vi "Meas Result Generate TWM InpZ Correction - Process Measurement.vi"(7 "table ref":refnum<vi>, 8 "error in":errorcluster, 11 "meas":T3={"swp cfg"={"N"=0, "R"=0, "f list"=[], "smpl delay"=0.0, "set delay"=0.0, "set delay np"=0.0, "meas root"=path "", "meas name"="", "meas a-index"=FALSE, "rnd sweep"=FALSE, "mode"=enum."Frequency", "swp mode"=enum."Linear", "avg"=0, "subrec"=0, "multi-freq"=FALSE, "selfcal"=FALSE, "selfcal period [h]"=0.0}, "bridge"={"type"=enum."TWM client", "TWM"={"pipe name"="", "parameters"=[], "handle"=0, "fixed aper [s]"=0.0, "f-list [Hz]"=[], "discrete f-list"=FALSE, "unc mode"=enum."None", "unc mcc"=0, "unc first"=FALSE, "alg id"=enum."TWM-LowZ - Low Z measurement"}, "last f"=0.0, "bias comp"={"bias type"=enum."dummy", "VISA"="", "Enable"=FALSE, "channel qu"=[], "channel Uinit"=[]}, "sim mode"=enum."Generic RLC network", "channel idns"=[], "sim phases"=1}, "src"={"type"=enum."Tektronix AFG3101C", "afg"={"VISA"="", "const"=0.0, "gen DC"=FALSE, "ext ref"=FALSE}, "cDAQ dds"={"device"="", "channels"=[], "mclk source"="", "mclk [Hz]"=0.0, "fs [Hz]"=0.0, "block [s]"=0.0, "buf [s]"=0.0, "task"="", "cmd queue"=refnum, "proc ref"=refnum, "smpl clock out"="/cDAQ3/PFI0", "export smpl clock"=FALSE, "DC ofs [V]"=[], "timebase source"="", "timebase mode"=enum."Local", "dither"=enum."Disabled", "dither level"=0.0}, "gain [V/A]"=1.0, "F5xxx session"={"VISA"="", "mode"=enum."AC voltage", "Earth on"=FALSE, "Ext ref lock"=FALSE}}, "results"=refnum} {"src"."cDAQ dds"."channels" min=0 step=1; "bridge"."TWM"."f-list [Hz]" format="%#_6p"; "swp cfg"."f list"."bias" format="%#_3p"; "swp cfg"."f list"."level" format="%#_3p"; "swp cfg"."f list"."fs [Hz]" format="%#_5p"; "swp cfg"."f list"."time [s]" format="%#_3p"; "swp cfg"."f list"."f/fs" format="%#_3p"; "swp cfg"."f list"."periods" format="%#_3f"; "swp cfg"."f list"."f [Hz]" format="%#_5p"}) -> (0 "error out":errorcluster, 3 "correction data":T1)   [LabVIEW 2020]
doc: "Generates input impedance correction matrix for TWM."
uses:
  meas session.ctl
  Meas Sweep Config.ctl
  Meas Freq Info.ctl
  meas_swp_mode.ctl
  meas_sweep_flist_mode.ctl
  bridge/Bridge Session.ctl
  bridge/Bridge Type.ctl
  drivers/TWM client/TWM Session.ctl
  drivers/TWM client/TWM parameters.ctl
  drivers/TWM client/Meas Proc QWTB Uncertainty Mode.ctl
  bridge/Bridge Algorithm.ctl
  bridge/Bridge Bias Session.ctl
  bridge/Bridge Bias Type.ctl
  bridge/Bridge Sim Mode.ctl
  source/Source Session.ctl
  source/Source Type.ctl
  drivers/AFG3101C/AFG3101C Session.ctl
  drivers/cDAQ DDS/cDAQ DDS Session.ctl
  drivers/cDAQ DDS/cDAQ DDS Setup.ctl
  drivers/cDAQ DDS/cDAQ DDS Timebase Mode.ctl
  drivers/cDAQ DDS/cDAQ DDS Dither.ctl
  drivers/Fluke 5XXX/top_lev/F5xxx_session.ctl
  drivers/Fluke 5XXX/top_lev/F5xxx_output_mode.ctl
  Meas Results Ref.ctl
  Meas Results.ctl
  bridge/Bridge Frequency Readings Data.ctl
  drivers/TWM client/Meas Proc QWTB Spectrum Data.ctl
  drivers/TWM client/TWM Phase Info.ctl
  Meas Results TWM Digitizer Correction Data.ctl
  Meas Results Correction Structuring Mode.ctl
  Meas Results Sweep Data Uncertainty Mode.ctl
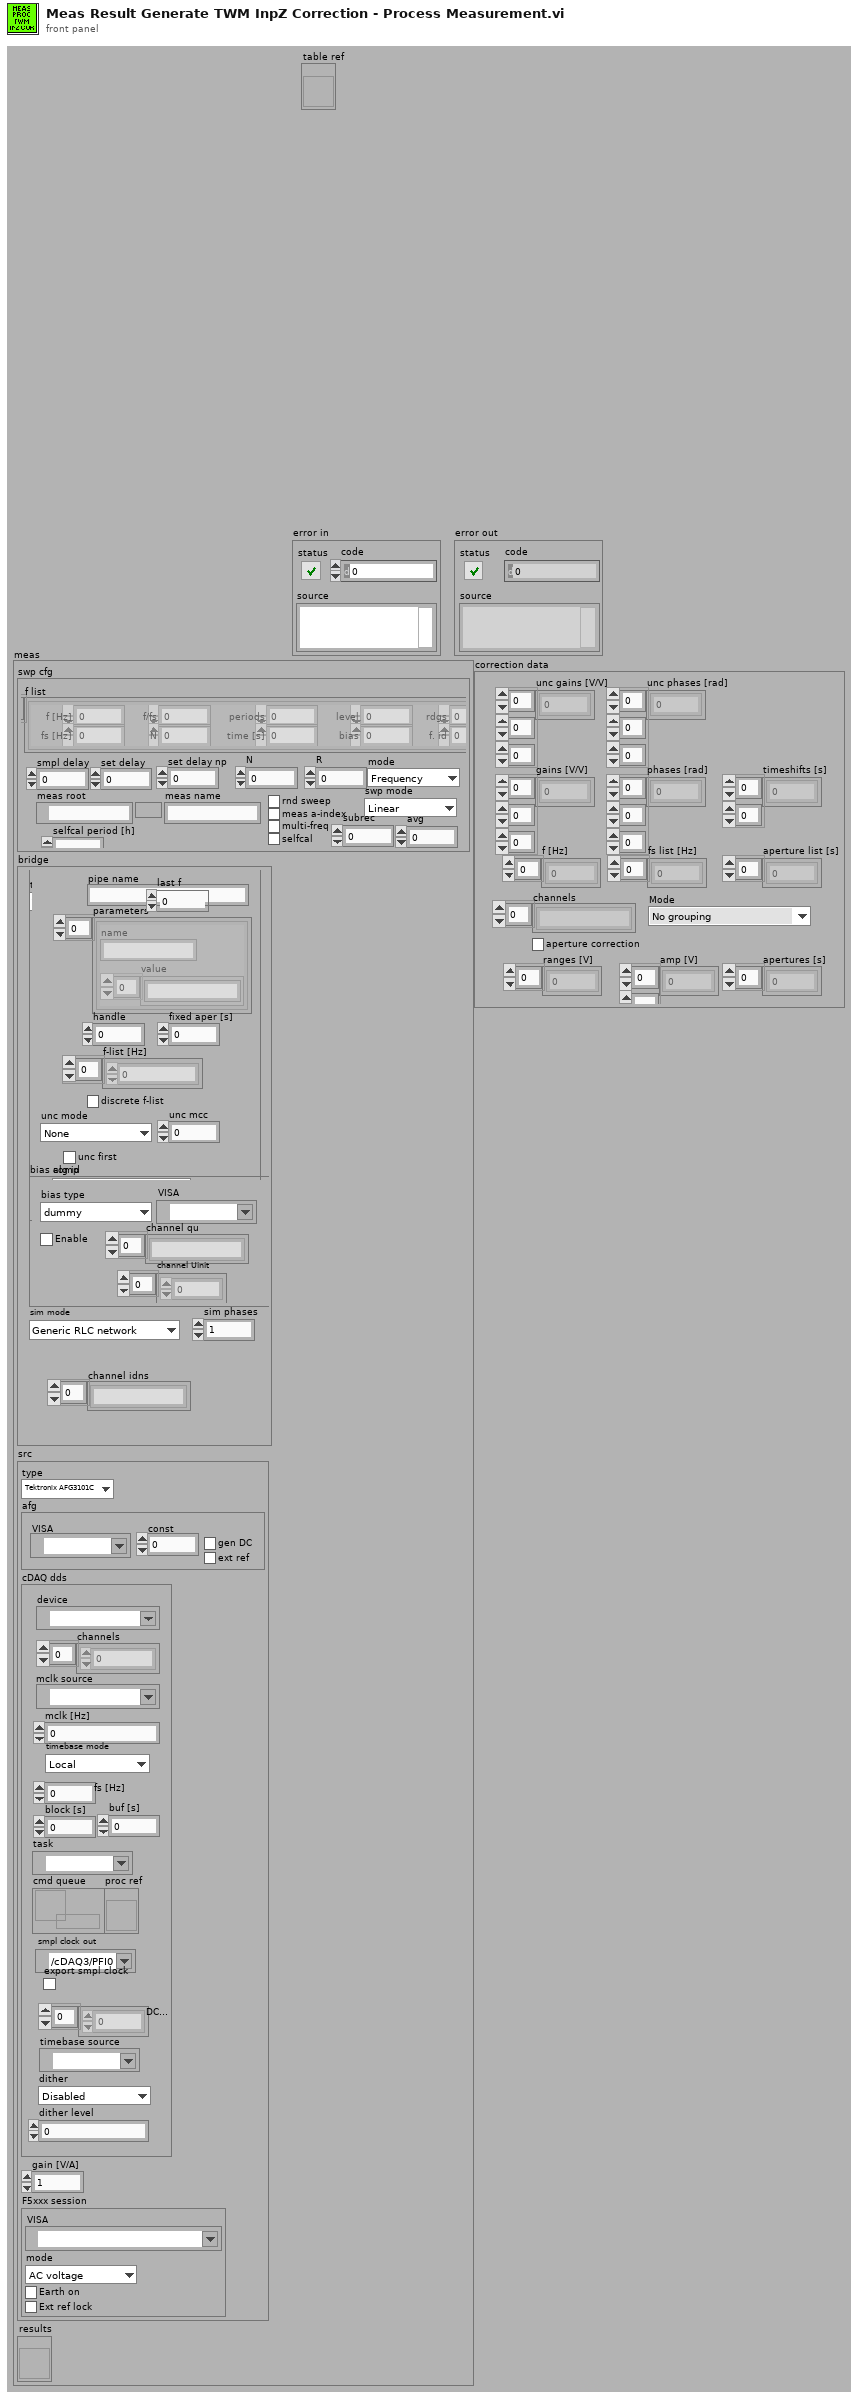
[diagram p1: front panel]
types:
  T1 = typedef "Meas Results TWM Digitizer Correction Data.ctl" = cluster{"gains [V/V]":dbl[][][], "phases [rad]":dbl[][][], "timeshifts [s]":dbl[][], "f [Hz]":dbl[], "fs list [Hz]":dbl[], "aperture list [s]":dbl[], "channels":string[], "Mode":T2, "aperture correction":bool, "ranges [V]":dbl[], "amp [V]":dbl[][], "apertures [s]":dbl[], "unc gains [V/V]":dbl[][][], "unc phases [rad]":dbl[][][]}
  T2 = typedef "Meas Results Correction Structuring Mode.ctl" = enum16{"No grouping", "Group by apertures (3458A)", "Group by fs (generic digitizer)"}
  T3 = typedef "meas session.ctl" = cluster{"swp cfg":T4, "bridge":T8, "src":T17, "results":T25}
  T4 = typedef "Meas Sweep Config.ctl" = cluster{"N":i32, "R":i32, "f list":T5[], "smpl delay":dbl, "set delay":dbl, "set delay np":dbl, "meas root":path, "meas name":string, "meas a-index":bool, "rnd sweep":bool, "mode":T6, "swp mode":T7, "avg":i32, "subrec":i32, "multi-freq":bool, "selfcal":bool, "selfcal period [h]":dbl}
  T5 = typedef "Meas Freq Info.ctl" = cluster{"f [Hz]":dbl, "periods":dbl, "f/fs":dbl, "time [s]":dbl, "fs [Hz]":dbl, "N":i32, "level":dbl, "bias":dbl, "rdgs":i32, "f. id":i32}
  T6 = typedef "meas_swp_mode.ctl" = enum16{"Frequency", "Level", "Bias"}
  T7 = typedef "meas_sweep_flist_mode.ctl" = enum16{"Linear", "Log10"}
  T8 = typedef "Bridge Session.ctl" = cluster{"type":T9, "TWM":T10, "last f":dbl, "bias comp":T14, "sim mode":T16, "channel idns":string[], "sim phases":i32}
  T9 = typedef "Bridge Type.ctl" = enum16{"TWM client", "dummy"}
  T10 = typedef "TWM Session.ctl" = cluster{"pipe name":string, "parameters":T11[], "handle":i32, "fixed aper [s]":dbl, "f-list [Hz]":dbl[], "discrete f-list":bool, "unc mode":T12, "unc mcc":i32, "unc first":bool, "alg id":T13}
  T11 = typedef "TWM parameters.ctl" = cluster{"name":string, "value":string[]}
  T12 = typedef "Meas Proc QWTB Uncertainty Mode.ctl" = enum16{"None", "GUF", "Monte Carlo"}
  T13 = typedef "Bridge Algorithm.ctl" = enum16{"TWM-LowZ - Low Z measurement", "TWM-InpZ - Digitizer input Z measurement"}
  T14 = typedef "Bridge Bias Session.ctl" = cluster{"bias type":T15, "VISA":refnum<visa-resource-name>, "Enable":bool, "channel qu":string[], "channel Uinit":dbl[]}
  T15 = typedef "Bridge Bias Type.ctl" = enum16{"dummy", "CMI LiBbias V1.0"}
  T16 = typedef "Bridge Sim Mode.ctl" = enum16{"Generic RLC network", "Interchannel transfer", "Input impedance"}
  T17 = typedef "Source Session.ctl" = cluster{"type":T18, "afg":T19, "cDAQ dds":T20, "gain [V/A]":dbl, "F5xxx session":T23}
  T18 = typedef "Source Type.ctl" = enum16{"Tektronix AFG3101C", "cDAQ DAC", "Fluke 5xxx", "Agilent 33120A", "dummy"}
  T19 = typedef "AFG3101C Session.ctl" = cluster{"VISA":refnum<visa-resource-name>, "const":dbl, "gen DC":bool, "ext ref":bool}
  T20 = typedef "cDAQ DDS Session.ctl" = cluster{"device":tag, "channels":i32[], "mclk source":tag, "mclk [Hz]":dbl, "fs [Hz]":dbl, "block [s]":dbl, "buf [s]":dbl, "task":refnum<k21>, "cmd queue":refnum<queue>, "proc ref":refnum<vi>, "smpl clock out":tag, "export smpl clock":bool, "DC ofs [V]":dbl[], "timebase source":tag, "timebase mode":T21, "dither":T22, "dither level":dbl}
  T21 = typedef "cDAQ DDS Timebase Mode.ctl" = enum16{"Local", "Take from ADC (e.g. NI 9238)", "Other source"}
  T22 = typedef "cDAQ DDS Dither.ctl" = enum16{"Disabled", "Gaussian"}
  T23 = typedef "F5xxx_session.ctl" = cluster{"VISA":refnum<visa-resource-name>, "mode":T24, "Earth on":bool, "Ext ref lock":bool}
  T24 = typedef "F5xxx_output_mode.ctl" = enum16{"AC voltage", "AC current"}
  T25 = typedef "Meas Results Ref.ctl" = refnum<vi>
  T26 = typedef "Meas Results Sweep Data Uncertainty Mode.ctl" = enum16{"ua(y)", "ua(y) (p=95%)", "uc(y) (p=95%)"}
  T27 = typedef "Meas Results.ctl" = cluster{"freqs":T28[][], "locked":bool, "last fid":i32, "modified":bool, "mjr name":string, "mnr name":string, "last spectra":T29[][], "saved?":bool, "TWM phase":T30[], "time start":timestamp, "time stop":timestamp}
  T28 = typedef "Bridge Frequency Readings Data.ctl" = cluster{"Udut":dbl[], "Iref":dbl[], "Udc":dbl[], "Idc":dbl[], "mjr":dbl[], "mnr":dbl[], "mjr_sh":dbl[], "mnr_sh":dbl[], "u(mjr)":dbl[], "u(mnr)":dbl[], "ua2(mjr)":dbl[], "ua2(mnr)":dbl[], "n":i32, "f [Hz]":dbl, "fs [Hz]":dbl, "aperture [s]":dbl}
  T29 = typedef "Meas Proc QWTB Spectrum Data.ctl" = cluster{"x":sgl[], "y":sgl[], "label":string}
  T30 = typedef "TWM Phase Info.ctl" = cluster{"ref chn id (I)":string, "dut chn id (U)":string, "ref chn range [V]":dbl, "dut chn range [V]":dbl, "aperture [s]":dbl, "fs [Hz]":dbl, "ref chn transducer (I)":string, "dut chn transducer (U)":string}
  T31 = typedef "Meas Results Sweep Data.ctl" = cluster{"Udut":dbl[], "Iref":dbl[], "Udc":dbl[], "Idc":dbl[], "mjr":dbl[], "mnr":dbl[], "mjr_sh":dbl[], "mnr_sh":dbl[], "f [Hz]":dbl[], "n [-]":i32[], "fs [Hz]":dbl[], "aperture [s]":dbl[]}
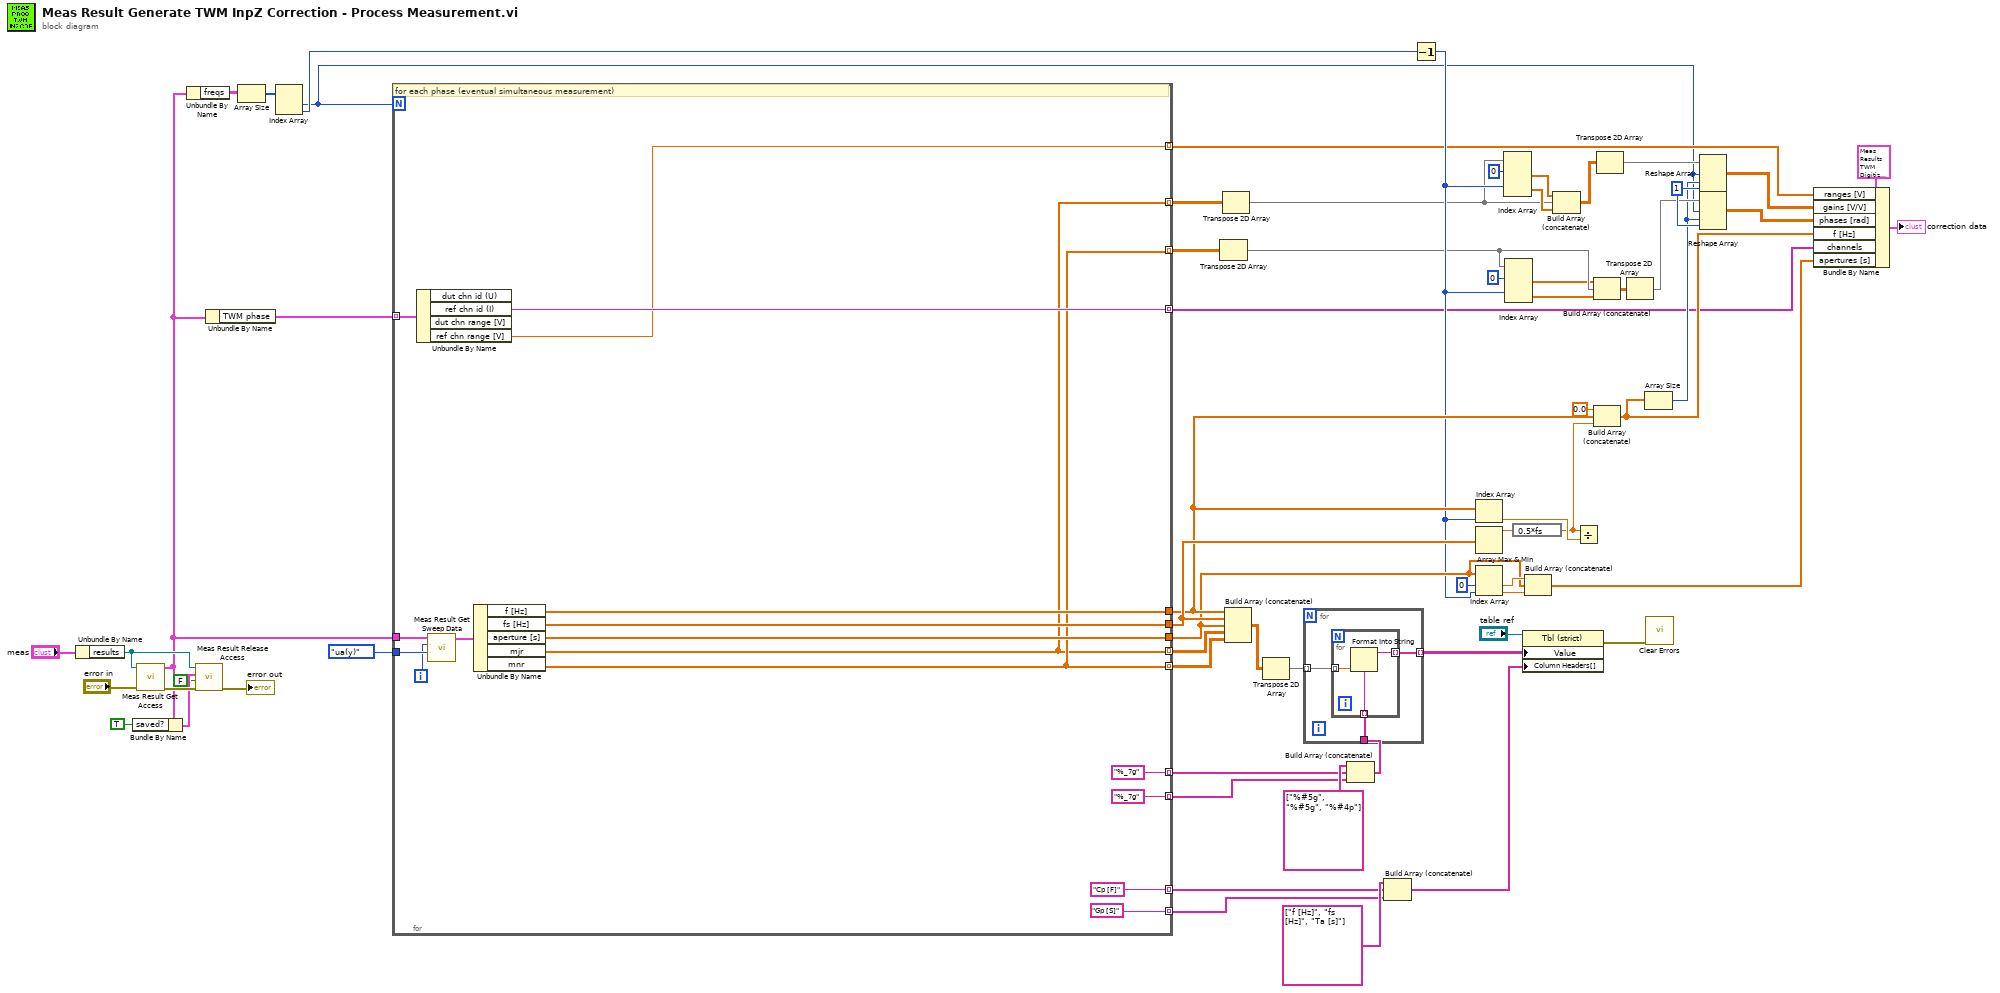
[diagram p0: block diagram]
diagram:
  w15 = 1 ("dimension size")
  n1 = Unbundle By Name("meas") -> ("results"=w59:T25)
  n2 = call "Meas Result Get Access.vi"("error in"="error in", "results ref"=w59) -> ("error out"=w62:errorcluster, "results data"=w47:T27)  [unwired: 8 in]
  n3 = Bundle By Name(cluster=w47, "saved?"=TRUE) -> (w60:T27)
  n4 = Unbundle By Name(w47) -> ("freqs"=w64:T28[][])
  n5 = call "Meas Result Release Access.vi"("error in"=w62, "Release only (True)"=FALSE, "results data in"=w60, "results ref"=w59) -> ("error out"=→"error out":errorcluster)  [unwired: 7 in]
  n6 = Unbundle By Name(w47) -> ("TWM phase"=w46:T30[])
  n7 = Array Size(array=w64) -> (size(s)=w63:i32[])
  n8 = Index Array(array=w63) -> (element #1=w5:i32, element #2=w16:i32)  [unwired: 2 in]
  n9 = for {
    N: w5 -> [_]
    tunnel: Meas_Results_Sweep_Data_Uncertainty_Mode."ua(y)" ("uncertainty mode") -> [w80]
    tunnel: w47 -> [w74]
    tunnel: [w79] -> w36
    tunnel: [w78] -> w40
    tunnel: [w77] -> w23
    tunnel: [w67] -> w53 mode=indexing
    tunnel: [w68] -> w52 mode=indexing
    tunnel: ["%_7g"] -> w50 mode=indexing
    tunnel: ["%_7g"] -> w49 mode=indexing
    tunnel: w46 -> [w73] mode=indexing
    tunnel: ["Cp [F]"] -> w32 mode=indexing
    tunnel: ["Gp [S]"] -> w31 mode=indexing
    tunnel: [w69] -> w9 mode=indexing
    tunnel: [w68] -> w8 mode=indexing
    tunnel: [w67] -> w7 mode=indexing
    tunnel: [w66] -> w6 mode=indexing
    i -> [w72]
    # "for each phase (eventual simultaneous measurement)"
    n10 = Unbundle By Name(w73) -> ("ref chn id (I)"=w69:string, "ref chn range [V]"=w66:dbl)  [unwired: 2 out]
    n11 = call "Meas Result Get Sweep Data.vi"("uncertainty mode"=w80, "phase index (default: 0)"=w72, "result"=w74) -> ("data"=w81:T31)  [unwired: 1 in, 2 out]
    n12 = Unbundle By Name(w81) -> ("f [Hz]"=w79:dbl[], "fs [Hz]"=w78:dbl[], "aperture [s]"=w77:dbl[], "mjr"=w67:dbl[], "mnr"=w68:dbl[])
  }
  n13 = Transpose 2D Array(2D array=w8) -> (transposed array=w3:dbl[][])
  n14 = Transpose 2D Array(2D array=w7) -> (transposed array=w4:dbl[][])
  n15 = Build Array (concatenate)(w36, w40, w23, w53, w52) -> (w54:dbl[][])
  n16 = Transpose 2D Array(2D array=w54) -> (transposed array=w55:dbl[][])
  n17 = Build Array (concatenate)(string[] ["%#5g", "%#5g", "%#4p"], w50, w49) -> (w48:string[])
  n18 = for {
    tunnel: w55 -> [w83] mode=indexing
    tunnel: w48 -> [w84]
    tunnel: [w82] -> w29 mode=indexing
    n19 = for {
      tunnel: w84 -> [w86] mode=indexing
      tunnel: w83 -> [w87] mode=indexing
      tunnel: [w85] -> w82 mode=indexing
      n20 = Format Into String(format string=w86, w87) -> (resulting string=w85:string)  [unwired: 2 in, 1 out]
    }
  }
  n21 = Build Array (concatenate)(string[] ["f [Hz]", "fs [Hz]", "Ta [s]"], w32, w31) -> (w28:string[])
  n22 = Decrement(x=w16) -> (x-1=w17:i32)
  n23 = Index Array(array=w36, index=w17) -> (element=w38:dbl)
  n24 = Array Max & Min(array=w40) -> (max value=w39:dbl)  [unwired: 3 out]
  n25 = Index Array(array=w23, index #1=0 ("index"), index #2=w17) -> (element #1=w25:dbl, element #2=w24:dbl)
  n26 = Index Array(array=w4, index (row) #1=0 ("index (row)"), index (row) #2=w17) -> (element #1=w43:dbl[], element #2=w42:dbl[])  [unwired: 2 in]
  n27 = Index Array(array=w3, index (row) #1=0 ("index (row)"), index (row) #2=w17) -> (element #1=w2:dbl[], element #2=w1:dbl[])  [unwired: 2 in]
  n28 = expression code="0.5*fs"(w39) -> (w35:dbl)
  n29 = property class="Tbl (strict)"(reference="table ref", "Value"=w29, "Column Headers[]"=w28) -> (error out=w27:errorcluster)  [unwired: 1 in, 1 out]
  n30 = Build Array (concatenate)(w25, w23, w24) -> (w22:dbl[])
  n31 = Build Array (concatenate)(w43, w4, w42) -> (w21:dbl[][])
  n32 = Divide(x=w35, y=w38) -> ()  [unwired: 1 out]
  n33 = Build Array (concatenate)(w2, w3, w1) -> (w18:dbl[][])
  n34 = Build Array (concatenate)(0.0 ("element"), w36, w35) -> (w12:dbl[])
  n35 = Transpose 2D Array(2D array=w21) -> (transposed array=w13:dbl[][])
  n36 = Transpose 2D Array(2D array=w18) -> (transposed array=w14:dbl[][])
  n37 = Array Size(array=w12) -> (size(s)=w11:i32)
  n38 = call <vilib>:"Clear Errors.vi"("error in (no error)"=w27) -> ()  [unwired: 5 in, 2 out]
  n39 = Reshape Array(w13, w5, w11, w15) -> (w20:dbl[][][])
  n40 = Reshape Array(w14, w5, w11, w15) -> (w19:dbl[][][])
  n41 = Bundle By Name(cluster=T1 {"gains [V/V]"=[], "phases [rad]"=[], "timeshifts [s]"=[], "f [Hz]"=[], "fs list [Hz]"=[], "aperture list [s]"=[], "channels"=[], "Mode"=enum."No grouping", "aperture correction"=FALSE, "ranges [V]"=[], "amp [V]"=[], "apertures [s]"=[], "unc gains [V/V]"=[], "unc phases [rad]"=[]} ("correction data"), "ranges [V]"=w6, "gains [V/V]"=w20, "phases [rad]"=w19, "f [Hz]"=w12, "channels"=w9, "apertures [s]"=w22) -> (→"correction data":T1)
